vi "OpenStratagem.vi"(11 "String":string) -> ()   [LabVIEW 2024]
uses:
  <vilib>/Utility/error.llb/Trim Whitespace One-Sided.vi
panel:
  in  "error in":errorcluster
  out "new picture":picture
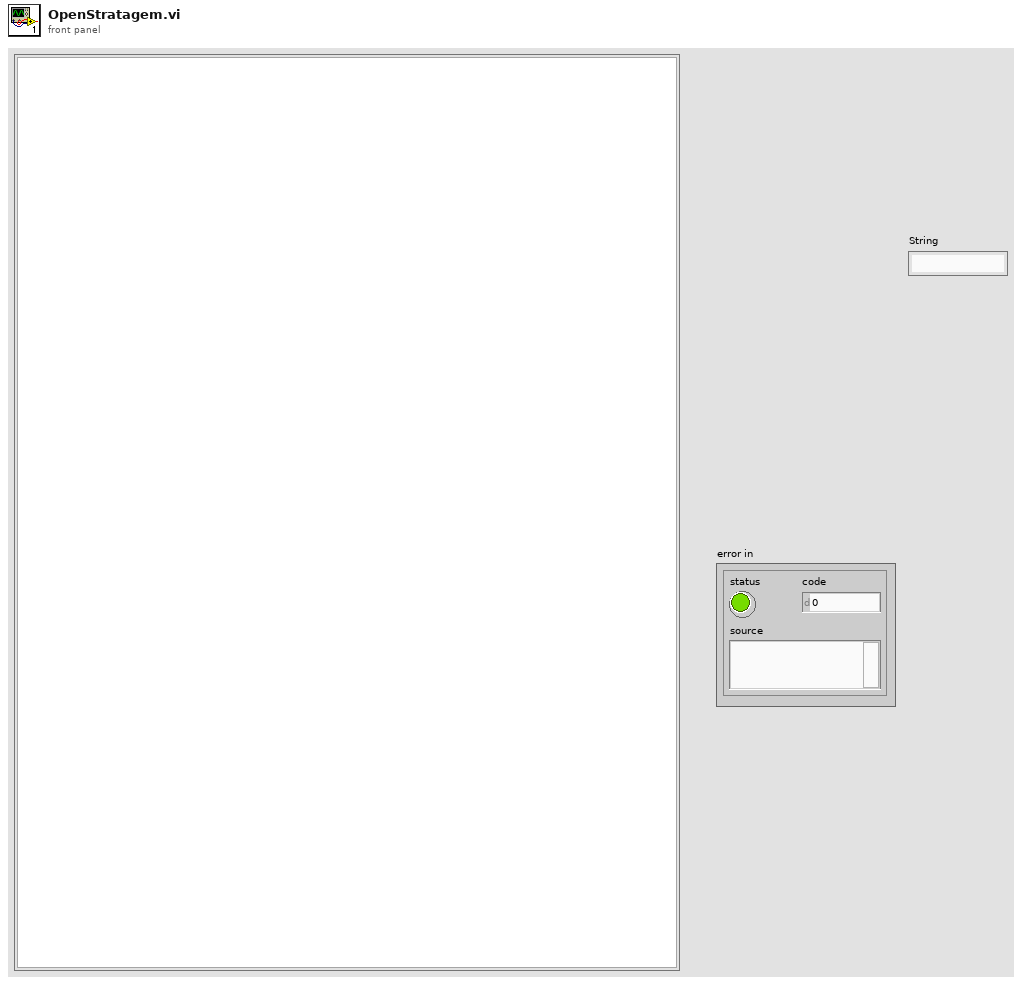
[diagram p1: front panel]
types:
  T1 = typedef "imagedata.ctl" = cluster{"image type":i32, "image depth":i32, "image":u8[], "mask":u8[], "colors":u32[], "Rectangle":cluster{"left":i16, "top":i16, "right":i16, "bottom":i16}}
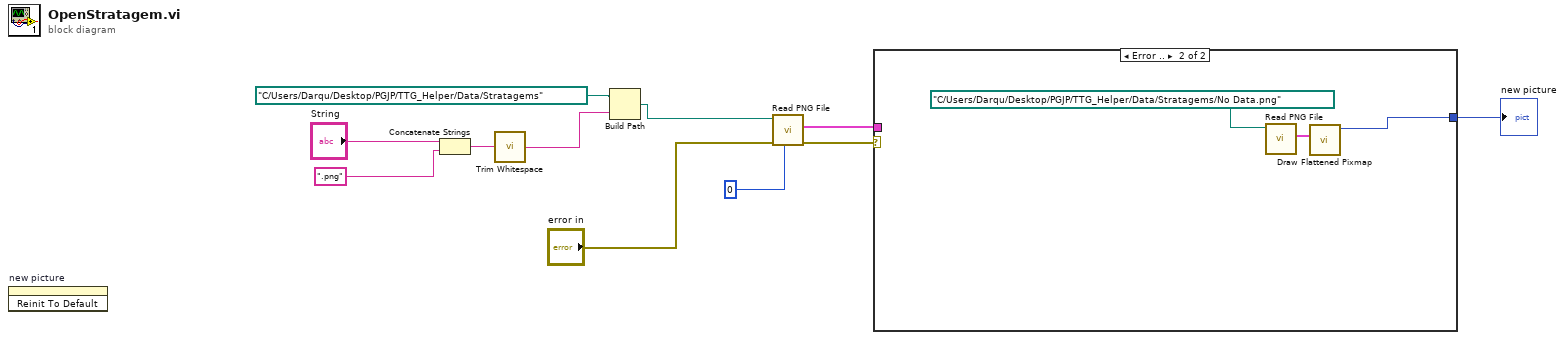
[diagram p0: block diagram]
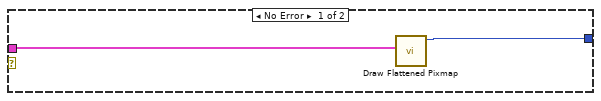
[diagram p2: hidden frame]
diagram:
  n1 = invoke on="new picture" class="Pict" method="Reinit To Default"() -> ()  [unwired: 3 in, 3 out]
  n2 = Concatenate Strings("String", ".png" ("string")) -> (w2:string)
  n3 = call <vilib>:"Trim Whitespace.vi"("string"=w2) -> ("trimmed string"=w1:string)  [unwired: 1 in]
  n4 = Build Path(base path=path "C:/Users/Darqu/Desktop/PGJP/TTG_Helper/Data/Stratagems", name or relative path=w1) -> (appended path=w7:path)
  n5 = call <vilib>:"Read PNG File.vi"("Transparency Thresh"=u8 0, "error in (no error)"="error in", "path to PNG file"=w7) -> ("error out"=w6:errorcluster, "image data"=w5:T1)  [unwired: 6 in, 1 out]
  n6 = case shown="Error .." w6 {
    tunnel: w5 -> [w13 _]
    tunnel: [w12 w14] -> w4
    frame No Error {
      n7 = call <vilib>:"Draw Flattened Pixmap.vi"("image data"=w13) -> ("new picture"=w12:picture)  [unwired: 8 in]
    }
    frame Error {
      n8 = call <vilib>:"Read PNG File.vi"("path to PNG file"=path "C:/Users/Darqu/Desktop/PGJP/TTG_Helper/Data/Stratagems/No Data.png") -> ("image data"=w16:T1)  [unwired: 8 in, 2 out]
      n9 = call <vilib>:"Draw Flattened Pixmap.vi"("image data"=w16) -> ("new picture"=w14:picture)  [unwired: 8 in]
    }
  }
  "new picture" <- w4
